vi "Close.vi"(2 "stop":refnum<vi>, 3 "error in":errorcluster, 4 "parent":refnum<vi>, 5 "subVI References":cluster{refnum<vi>[], refnum<vi>[]}) -> (0 "error out":errorcluster)   [LabVIEW 2020]
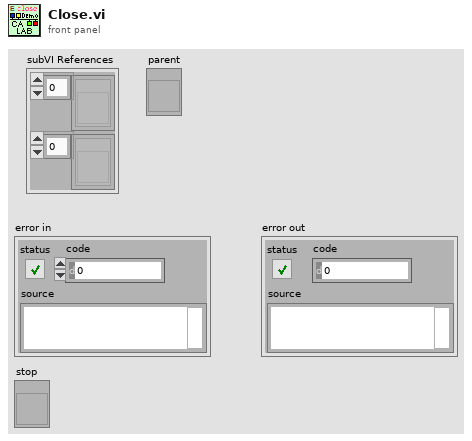
[diagram p1: front panel]
types:
  T1 = enum8{"Enabled", "Disabled", "Disabled and Grayed Out"}
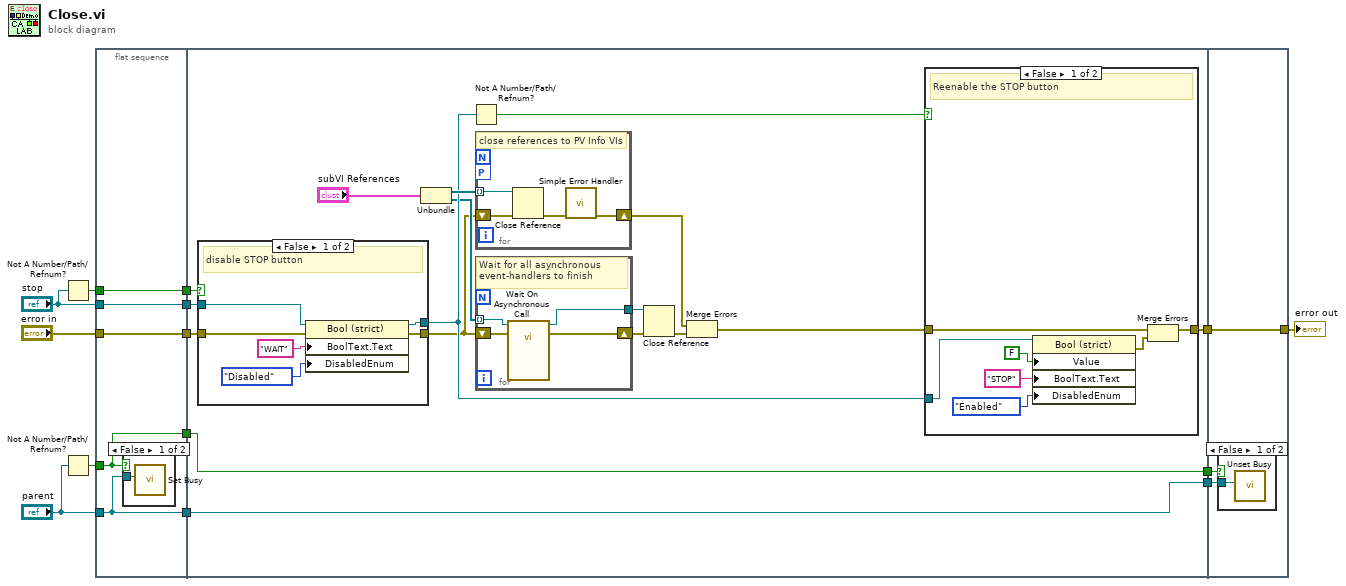
[diagram p0: block diagram]
diagram:
  n1 = Not A Number/Path/Refnum?(number/path/refnum="stop") -> (NaN/Path/Refnum?=w12:bool)
  n2 = Not A Number/Path/Refnum?(number/path/refnum="parent") -> (NaN/Path/Refnum?=w5:bool)
  n3 = flat-sequence {
    tunnel: "stop" -> [w17]
    tunnel: w12 -> [w18]
    tunnel: "error in" -> [w19]
    tunnel: [w19] -> w10
    tunnel: [w18] -> w9
    tunnel: [w17] -> w8
    tunnel: "parent" -> [w16]
    tunnel: [w16] -> w6
    tunnel: w5 -> [w15]
    tunnel: [w15] -> w2
    tunnel: w10 -> [w35]
    tunnel: w9 -> [w34]
    tunnel: w8 -> [w32]
    tunnel: [w37] -> w7
    tunnel: w6 -> [w22]
    tunnel: [w22] -> w3
    tunnel: w2 -> [w21]
    tunnel: [w21] -> w1
    tunnel: [w64] -> w14
    tunnel: w7 -> [w64]
    tunnel: w3 -> [w63]
    tunnel: w1 -> [w62]
    frame #0 {
      n4 = case shown="False" w15 {
        tunnel: w16 -> [w20 _]
        frame False {
          n5 = call <vilib>:"Set Busy.vi"("VI reference (current VI)"=w20) -> ()  [unwired: 9 in, 2 out]
        }
        frame True {
        }
      }
    }
    frame #1 {
      n6 = case shown="False" w34 {
        tunnel: [w53 w57] -> w28
        tunnel: w35 -> [w52 w57]
        tunnel: w32 -> [w51 w56]
        tunnel: [w50 w56] -> w31
        frame False {
          # "disable STOP button"
          n7 = property class="Bool (strict)"(reference=w51, error in=w52, "BoolText.Text"="WAIT" ("Boolean Text.Text"), "DisabledEnum"=T1."Disabled" ("Disabled")) -> (reference out=w50:refnum<vi>, error out=w53:errorcluster)
        }
        frame True {
        }
      }
      n8 = Unbundle("subVI References") -> (w36:refnum<vi>[], w29:refnum<vi>[])
      n9 = Not A Number/Path/Refnum?(number/path/refnum=w31) -> (NaN/Path/Refnum?=w33:bool)
      n10 = for {
        shift-right: [w58] -> w27
        shift-left: w28 -> [w61]
        tunnel: w36 -> [w59] mode=indexing
        workers-P: _ -> [_]
        # "close references to PV Info VIs"
        n11 = Close Reference(reference=w59, error in (no error)=w61) -> (error out=w60:errorcluster)
        n12 = call <vilib>:"Simple Error Handler.vi"("error in (no error)"=w60) -> ("error out"=w58:errorcluster)  [unwired: 4 in, 4 out]
      }
      n13 = for {
        tunnel: w29 -> [w41] mode=indexing
        shift-right: [w39] -> w25
        shift-left: w28 -> [w40]
        tunnel: [w38] -> w23
        # "Wait for all asynchronous event-handlers to finish"
        n14 = call-by-ref "Wait On Asynchronous Call"(reference=w41, error in=w40) -> (reference out=w38:refnum<vi>, error out=w39:errorcluster)  [unwired: 12 in]
      }
      n15 = Close Reference(reference=w23, error in (no error)=w25) -> (error out=w24:errorcluster)
      n16 = Merge Errors(w27, w24) -> (w26:errorcluster)
      n17 = case shown="False" w33 {
        tunnel: w26 -> [w44 w49]
        tunnel: [w42 w49] -> w37
        tunnel: w31 -> [w45 _]
        frame False {
          # "Reenable the STOP button"
          n18 = property class="Bool (strict)"(reference=w45, "Value"=FALSE, "BoolText.Text"="STOP" ("Label.Text"), "DisabledEnum"=T1."Enabled" ("Disabled")) -> (error out=w43:errorcluster)  [unwired: 1 in, 1 out]
          n19 = Merge Errors(w44, w43) -> (w42:errorcluster)
        }
        frame True {
        }
      }
    }
    frame #2 {
      n20 = case shown="False" w62 {
        tunnel: w63 -> [w65 _]
        frame False {
          n21 = call <vilib>:"Unset Busy.vi"("VI reference (current VI)"=w65) -> ()  [unwired: 10 in, 1 out]
        }
        frame True {
        }
      }
    }
  }
  "error out" <- w14
